vi "Read DAQ FIFO Direct Dispatch.vi"(7 "Release Lock":bool=TRUE, 8 "error in (no error)":errorcluster, 9 "Timeout (ms)":i32=100, 10 "DAQ In":T1[](array[typedef]), 11 "CIFTag in":refnum<class "CIFChannels.lvclass">) -> (0 "error out":errorcluster, 1 "timed out?":bool, 2 "DAQ Out":T1[](array[typedef]), 3 "CIFTag out":refnum<class "CIF_NIChn_Fifo_DAQ.lvclass">, 4 "Header":T2)   [LabVIEW 2021, in "CIF_NIChn_Fifo_DAQ.lvclass"]
uses:
  CIF_NIChn_Fifo_DAQ.lvclass
  CIF_NIChn_Fifo_DAQ.lvclass/CIF_NIChn_Fifo_DAQ.ctl
  ChannelCommon/typedef/FIFO Header.ctl
  ChannelCommon/ChannelCommon.lvlib
  ChannelCommon/typedef/Datatype Waveform.ctl
  CIFChannels/CIFChannels.lvclass
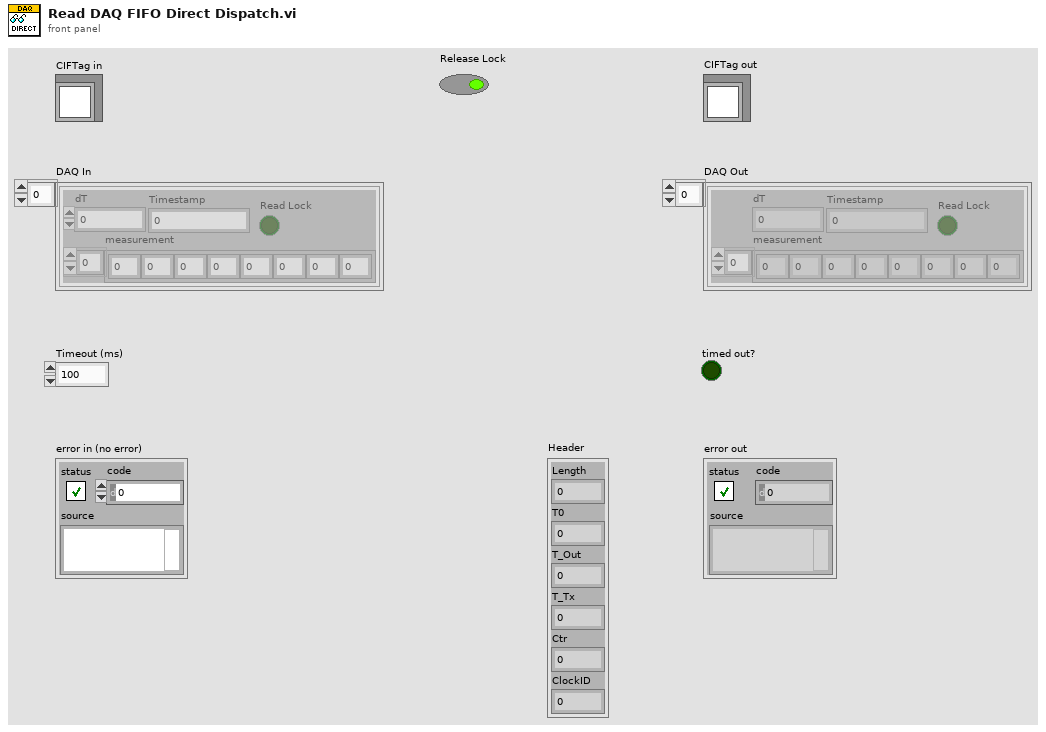
[diagram p1: front panel]
types:
  T1 = typedef "ChannelCommon.lvlib/Datatype Waveform.ctl" = cluster{"measurement":dbl[], "dT":dbl, "Timestamp":u64, "Read Lock":bool}
  T2 = typedef "ChannelCommon.lvlib/FIFO Header.ctl" = cluster{"Length":u64, "T0":u64, "T_Out":u64, "T_Tx":u64, "Ctr":u64, "ClockID":u8}
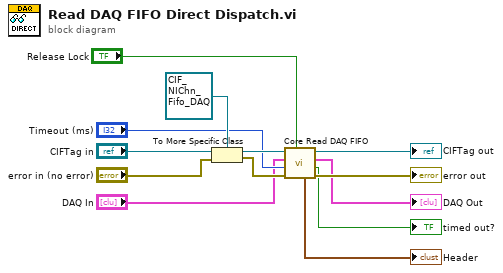
[diagram p0: block diagram]
diagram:
  n1 = To More Specific Class(target class=refnum<class "CIF_NIChn_Fifo_DAQ.lvclass"> refnum ("CIFTag in"), reference="CIFTag in", error in="error in (no error)") -> (specific class reference=w10:refnum<class "CIF_NIChn_Fifo_DAQ.lvclass">, error out=w9:errorcluster)
  n2 = call "Core Read DAQ FIFO.vi"("Release Lock"="Release Lock", "error in (no error)"=w9, "Timeout (ms)"="Timeout (ms)", "DAQ In"="DAQ In", "CIFTag in"=w10) -> ("error out"=→"error out":errorcluster, "timed out?"=→"timed out?":bool, "DAQ Out"=→"DAQ Out":T1[], "CIFTag out"=→"CIFTag out":refnum<class "CIF_NIChn_Fifo_DAQ.lvclass">, "Header"=→"Header":T2)  [unwired: 2 in]
